vi "PH_Beckhoff_StepMot.declare analog InputTags.vi"(3 "Instance Name":string="N/A") -> (0 "Analog Inputs":T1, 1 "Description":string)   [LabVIEW 2014, in "PH_Beckhoff_StepMot.lvlib"]
uses:
  PH_Beckhoff_StepMot.lvlib
  PH_Beckhoff/PH_Beckhoff.Analog Inputs.ctl
  PH_Beckhoff/PH_Beckhoff.Scaling Type.ctl
  PH_Beckhoff_StepMot.Force Sensor Tags.ctl
  PH_Beckhoff_StepMot.Force Sensor Location.ctl
  PH_Beckhoff/PH_Beckhoff.lvlib
panel:
  out "Right Size?":bool
  # "Let this VI run to check the size!"
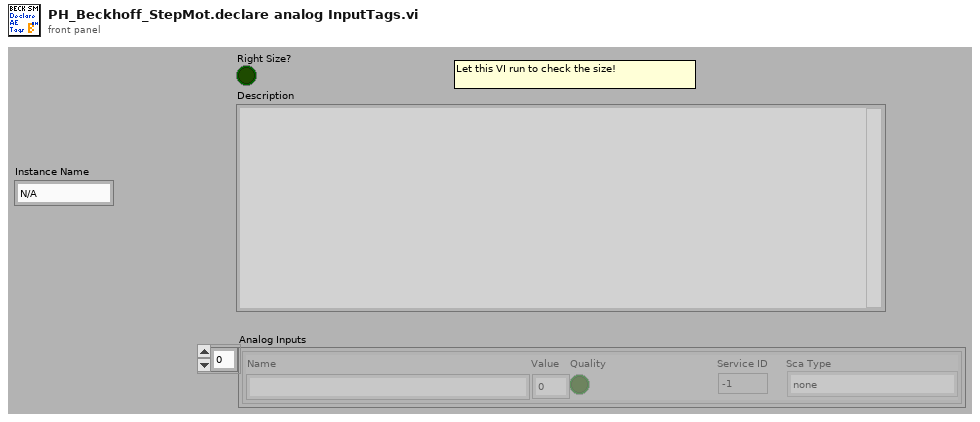
[diagram p1: front panel]
types:
  T1 = typedef "PH_Beckhoff.lvlib/PH_Beckhoff.Analog Inputs.ctl" = cluster{"Name":string, "Value":u32, "Quality":bool, "Service ID":i32, "Sca Type":T2}[]
  T2 = typedef "PH_Beckhoff.lvlib/PH_Beckhoff.Scaling Type.ctl" = enum16{"none", "0 ... 15 Bit -> 0 ... 5", "0 ... 15 Bit -> 0 ... 10", "0 ... 15 Bit -> 0 ... 25", "0 ... 15 Bit -> 4 ... 20", "0 ... 15 Bit -> 0 ... 1", "0 ... 15 Bit -> 0 ... 20000", "0 ... 15 Bit -> 0 ... 24000"}
  T3 = cluster{"Name":string, "Value":u32, "Quality":bool, "Service ID":i32, "Sca Type":T2}
  T4 = typedef "PH_Beckhoff_StepMot.lvlib/PH_Beckhoff_StepMot.Force Sensor Location.ctl" = enum16{"no Info", "MM1"}
  T5 = typedef "PH_Beckhoff_StepMot.lvlib/PH_Beckhoff_StepMot.Force Sensor Tags.ctl" = enum16{"top-front", "top-back", "bottom-front", "bottom-back"}
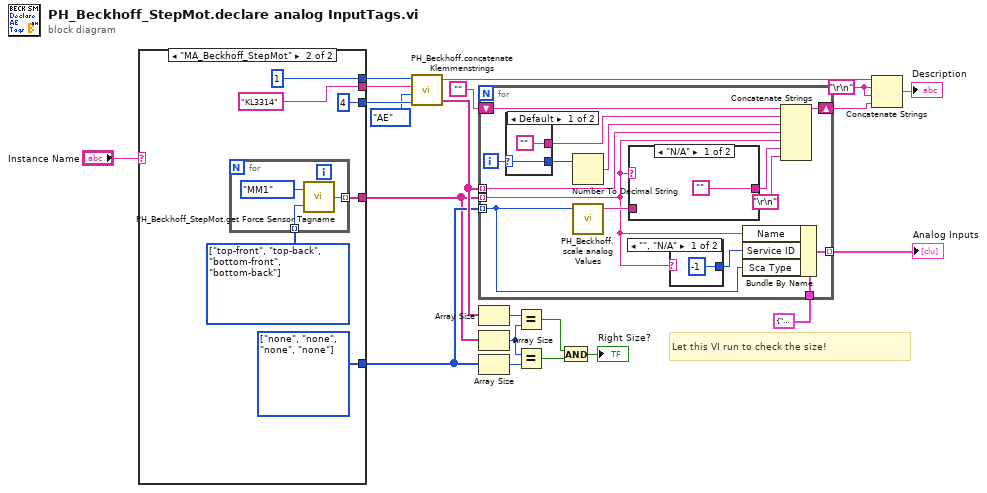
[diagram p0: block diagram]
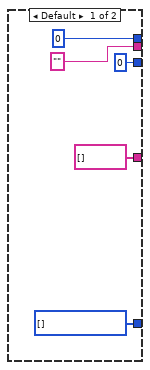
[diagram p2: hidden frame]
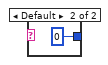
[diagram p3: hidden frame]
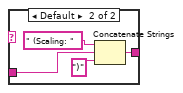
[diagram p4: hidden frame]
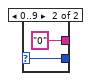
[diagram p5: hidden frame]
diagram:
  w19 = "\r\n"
  # "Let this VI run to check the size!"
  n1 = case shown="\"MA_Beckhoff_StepMot\"" "Instance Name" {
    tunnel: ["" ("Klemmenname") "KL3314" ("Klemmenname")] -> w15
    tunnel: [0 ("# of In- or Outputs") 4 ("# of In- or Outputs")] -> w14
    tunnel: [0 ("Quantity") 1 ("Quantity")] -> w9
    tunnel: [w24 w30] -> w4
    tunnel: [string[] [] w28] -> w3
    frame Default {
      w24 = T2[] [] items=["none", "0 ... 15 Bit -> 0 ... 5", "0 ... 15 Bit -> 0 ... 10", "0 ... 15 Bit -> 0 ... 25", "0 ... 15 Bit -> 4 ... 20", "0 ... 15 Bit -> 0 ... 1", "0 ... 15 Bit -> 0 ... 20000", "0 ... 15 Bit -> 0 ... 24000"]
    }
    frame "MA_Beckhoff_StepMot" {
      w27 = T5[] [enum."top-front", enum."top-back", enum."bottom-front", enum."bottom-back"] items=["top-front", "top-back", "bottom-front", "bottom-back"]
      w30 = T2[] [enum."none", enum."none", enum."none", enum."none"] items=["none", "0 ... 15 Bit -> 0 ... 5", "0 ... 15 Bit -> 0 ... 10", "0 ... 15 Bit -> 0 ... 25", "0 ... 15 Bit -> 4 ... 20", "0 ... 15 Bit -> 0 ... 1", "0 ... 15 Bit -> 0 ... 20000", "0 ... 15 Bit -> 0 ... 24000"]
      n2 = for {
        tunnel: [w35] -> w28 mode=indexing
        tunnel: w27 -> [w33] mode=indexing
        n3 = call "PH_Beckhoff_StepMot.get Force Sensor Tagname.vi"("Force Sensor Tag"=w33, "Force Sensor Location"=PH_Beckhoff_StepMot.Force_Sensor_Location."MM1") -> ("Force Sensor Tagname"=w35:string)
      }
    }
  }
  n4 = call "PH_Beckhoff.concatenate Klemmenstrings.vi"("# of In- or Outputs"=w14, "Type"=enum16{"AE", "AA", "DE", "DA", "SE"}."AE", "Klemmenname"=w15, "Quantity"=w9) -> ("concatenated string array"=w7:string[], "\"<Type>: <Quantity> x <Klemmenname>\""=w8:string)  [unwired: 1 out]
  n5 = for {
    tunnel: w3 -> [w36] mode=indexing
    tunnel: w7 -> [w46] mode=indexing
    shift-right: [w39] -> w20
    shift-left: "" -> [w40]
    tunnel: w4 -> [w37] mode=indexing
    tunnel: T3 {"Name"="", "Value"=0, "Quality"=FALSE, "Service ID"=0, "Sca Type"=enum."none"} ("Analog Input Value") -> [w44]
    tunnel: [w45] -> w6 mode=indexing
    i -> [w50]
    n6 = case shown="Default" w50 {
      selector: w50 -> [w58 w61]
      tunnel: [w58 w61] -> w49
      tunnel: ["" "0"] -> w48
      frame Default {
      }
      frame 0..9 {
      }
    }
    n7 = Number To Decimal String(number=w49) -> (decimal integer string=w47:string)  [unwired: 1 in]
    n8 = call "PH_Beckhoff.scale analog Values.vi"("Sca Type"=w37) -> ("Scaling"=w43:string)  [unwired: 2 in, 2 out]
    n9 = case shown="\"N/A\"" w36 {
      tunnel: w43 -> [_ w56]
      tunnel: ["" w54] -> w42
      frame "N/A" {
      }
      frame Default {
        n10 = Concatenate Strings(" (Scaling: " ("string"), w56, ")" ("string")) -> (w54:string)
      }
    }
    n11 = case shown="\"\", \"N/A\"" w36 {
      tunnel: [-1 0] -> w38
      frame "", "N/A" {
      }
      frame Default {
      }
    }
    n12 = Bundle By Name(cluster=w44, "Name"=w36, "Service ID"=w38, "Sca Type"=w37) -> (w45:T3)
    n13 = Concatenate Strings(w40, w48, w47, w46, w36, w42, "\r\n") -> (w39:string)
  }
  "Analog Inputs" <- w6
  n14 = Array Size(array=w7) -> (size(s)=w17:i32)
  n15 = Array Size(array=w3) -> (size(s)=w13:i32)
  n16 = Array Size(array=w4) -> (size(s)=w12:i32)
  n17 = Equal?(x=w17, y=w13) -> (x = y?=w16:bool)
  n18 = Equal?(x=w13, y=w12) -> (x = y?=w10:bool)
  n19 = And(x=w16, y=w10) -> (x .and. y?=→"Right Size?":bool)
  n20 = Concatenate Strings(w8, w19, w19, w20) -> (→"Description":string)
